vi "_TangoAttributeDataReadyEventHandler.vi"(3 "error in":errorcluster, 4 "timeout (ms)":i32=1000, 5 "attribute data ready event ref":T2) -> (0 "error out":errorcluster, 1 "attribute data ready":T1, 2 "event timeout":bool)   [LabVIEW 2014, in "tango.lvlib"]
uses:
  tango.lvlib
  Common VIs/Typedefs/_AttributeDataReadyEventRef.ctl
  Private VIs/Events/_AttributeDataReady_t.ctl
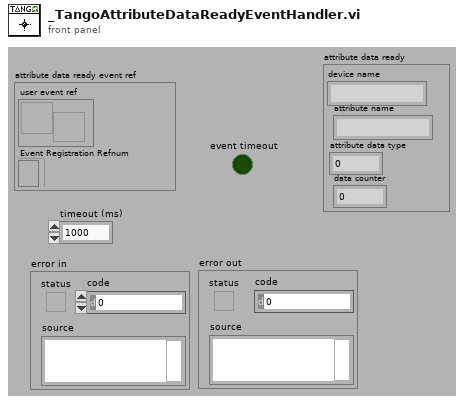
[diagram p1: front panel]
types:
  T1 = typedef "tango.lvlib/_AttributeDataReady_t.ctl" = cluster{"device name":string, "attribute name":string, "attribute data type":i16, "data counter":i16}
  T2 = typedef "tango.lvlib/_AttributeDataReadyEventRef.ctl" = cluster{"user event ref":refnum<user-event>, "user event reg refnum":refnum<event-registration>}
  T3 = cluster{"device name":string, "attribute name":string, "attribute data type":i16, "data counter":i16}
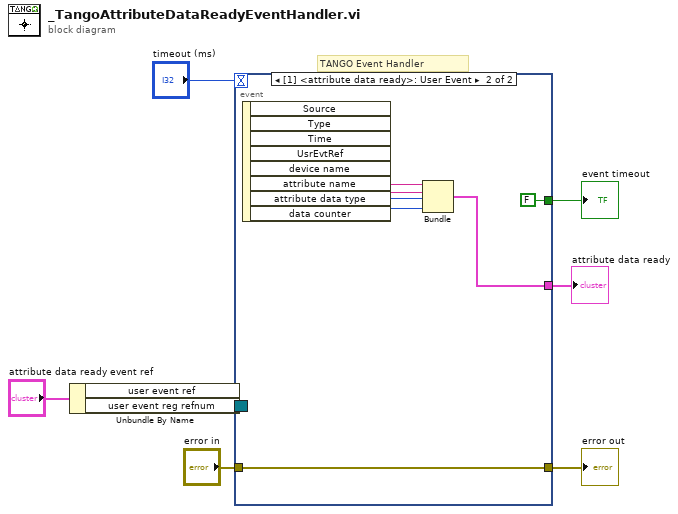
[diagram p0: block diagram]
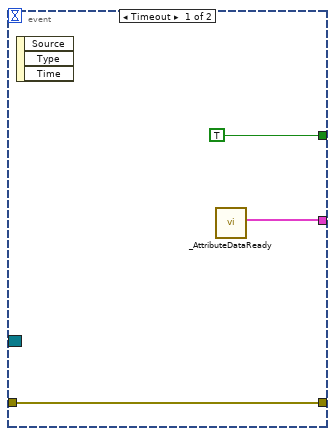
[diagram p2: hidden frame]
diagram:
  # "TANGO Event Handler"
  n1 = Unbundle By Name("attribute data ready event ref") -> ("user event reg refnum"=w3:refnum<event-registration>)  [unwired: 1 out]
  n2 = event shown="[1] <attribute data ready>: User Event" {
    selector: w3 -> [_ _]
    dyn-events: _ -> [_ _]
    timeout: "timeout (ms)" -> [_ _]
    tunnel: [TRUE FALSE] -> w7
    tunnel: "error in" -> [w9 w11]
    tunnel: [w9 w11] -> w5
    tunnel: [w8 w12] -> w1
    event Timeout {
      n3 = event-data() -> ()  [unwired: 1 in, 3 out]
      n4 = call "_AttributeDataReady.vi"() -> ("attribute data ready"=w8:T1)
    }
    event User Event {
      n5 = event-data() -> ("device name"=w16:string, "attribute name"=w15:string, "attribute data type"=w14:i16, "data counter"=w13:i16)  [unwired: 1 in, 4 out]
      n6 = Bundle("device name"=w16, "attribute name"=w15, "attribute data type"=w14, "data counter"=w13) -> (w12:T3)  [unwired: 1 in]
    }
  }
  "event timeout" <- w7
  "error out" <- w5
  "attribute data ready" <- w1
